vi "全局 所有参数.vi"() -> ()   [LabVIEW 2016]
panel:
  in  "总磷加标回收率":string[][](array[string])
  in  "总氮加标回收率":string[][](array[string])
  in  "氨氮加标回收率":string[][](array[string])
  in  "CODCr加标回收率":string[][](array[string])
  in  "CODMn加标回收率":string[][](array[string])
  in  "累积流量":string[][](array[string])
  in  "瞬时流量":string[][](array[string])
  in  "流速":string[][](array[string])
  in  "水位":string[][](array[string])
  in  "盐度":string[][](array[string])
  in  "铜":string[][](array[string])
  in  "藻密度":string[][](array[string])
  in  "叶绿素":string[][](array[string])
  in  "浊度":string[][](array[string])
  in  "DO":string[][](array[string])
  in  "水温":string[][](array[string])
  in  "电导率":string[][](array[string])
  in  "总磷":string[][](array[string])
  in  "总氮":string[][](array[string])
  in  "CODMn":string[][](array[string])
  in  "氨氮":string[][](array[string])
  in  "CODCr":string[][](array[string])
  in  "PH":string[][](array[string])
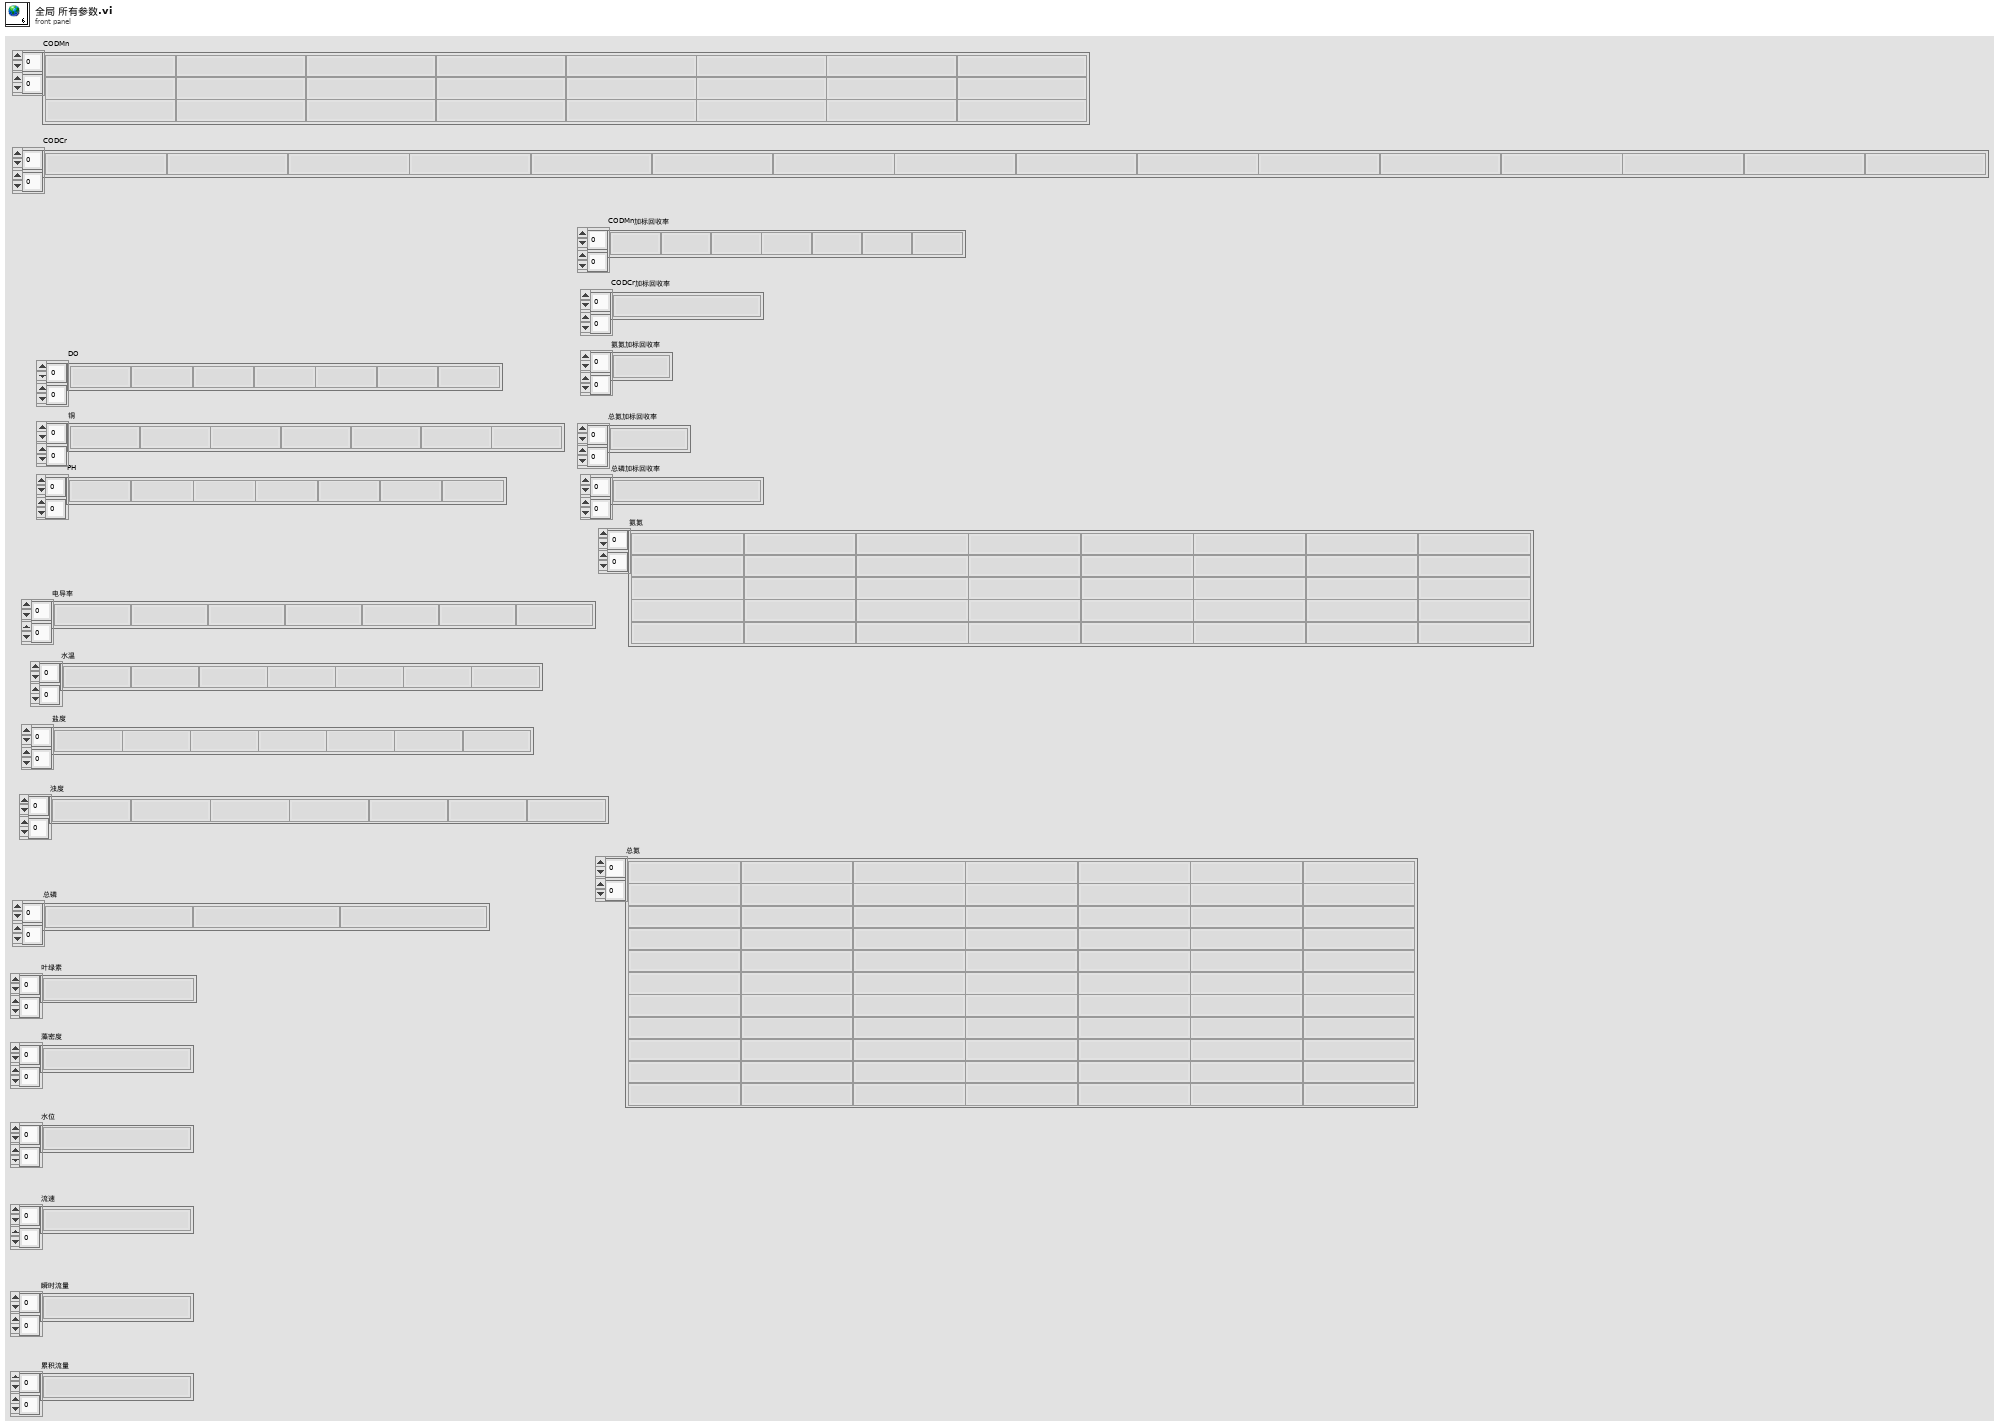
[diagram p1: front panel]
diagram:
